vi "Wait_Seconds_with_display_Simple.vi"(2 "Message":string, 3 "Seconds to wait":dbl=1.0 format="%.2f") -> (1 "Stopped":bool)   [LabVIEW 2021]
doc: "Waits the number of seconds specified by the Seconds to Wait input, divided by the time dilation factor, if used."
uses:
  Globals/Meas_global.vi
panel:
  in  "stop":bool
  out "Seconds waited":u32(slide) scale=0.0..60.0
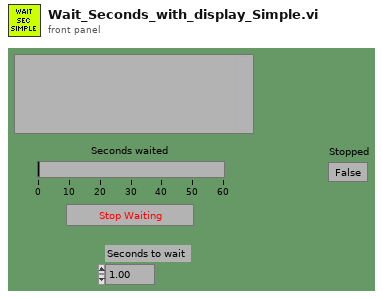
[diagram p1: front panel]
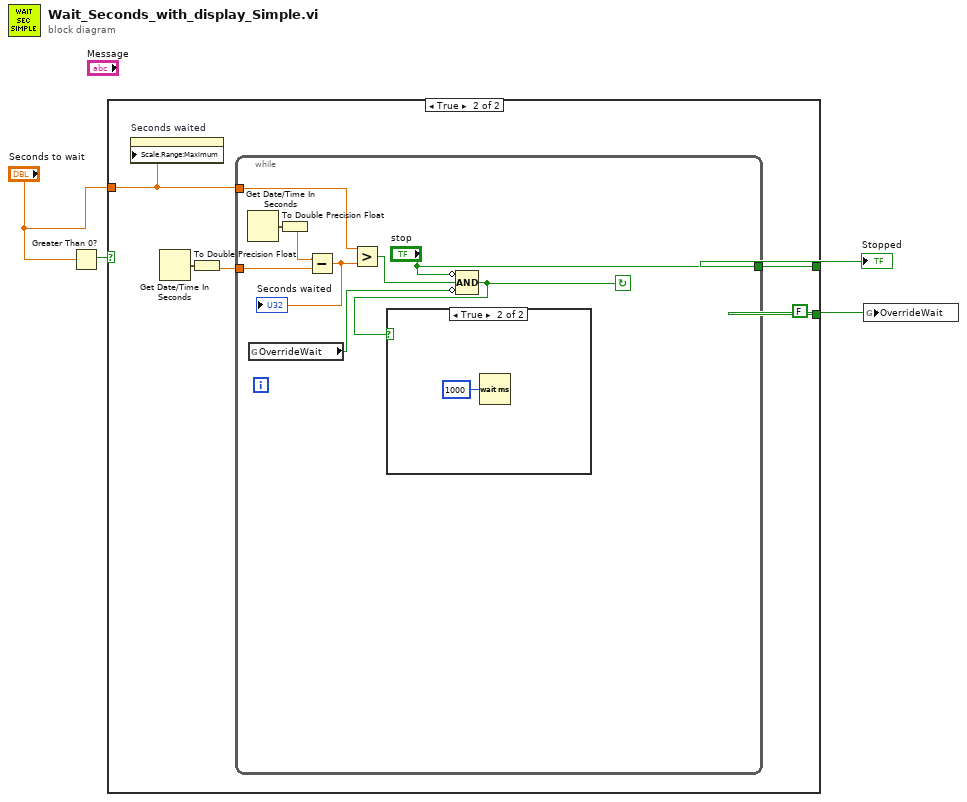
[diagram p0: block diagram]
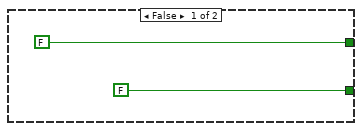
[diagram p2: hidden frame]
diagram:
  n1 = Greater Than 0?(x="Seconds to wait") -> (x > 0?=w3:bool)
  n2 = case shown="True" w3 {
    tunnel: [FALSE ("stop") w11] -> w4
    tunnel: "Seconds to wait" -> [_ w9]
    tunnel: [FALSE FALSE] -> w1
    frame False {
    }
    frame True {
      n3 = property on="Seconds waited" class="Slide (strict)"("Scale.Range:Maximum"=w9) -> ()  [unwired: 2 in, 2 out]
      n4 = Get Date/Time In Seconds() -> (seconds since 1Jan1904=w8:timestamp)
      n5 = To Double Precision Float(number=w8) -> (double precision float=w10:dbl)
      n6 = while {
        tunnel: ["stop"] -> w11
        tunnel: w9 -> [w17]
        tunnel: w10 -> [w20]
        stop <- w13 continue-if-true
        n7 = Get Date/Time In Seconds() -> (seconds since 1Jan1904=w14:timestamp)
        n8 = global read "Meas_global.vi" "OverrideWait"() -> (w12:bool)
        n9 = To Double Precision Float(number=w14) -> (double precision float=w15:dbl)
        n10 = Subtract(x=w15, y=w20) -> (x-y=w16:dbl)
        "Seconds waited" <- w16
        n11 = Greater?(x=w17, y=w16) -> (0:w19:bool)
        n12 = Compound Arithmetic op=AND(invert "stop", w19, invert w12) -> (w13:bool)
        n13 = case shown="True" w13 {
          frame False {
          }
          frame True {
            n14 = Wait (ms)(milliseconds to wait=u32 1000) -> ()  [unwired: 1 out]
          }
        }
      }
    }
  }
  "Stopped" <- w4
  n15 = global write "Meas_global.vi" "OverrideWait"(w1) -> ()
